vi "get Rx Packet Error.vi"(8 "error in (no error)":errorcluster, 10 "error":u8, 11 "protocol_version":i32) -> (0 "error out":errorcluster, 3 "function return":string)   [LabVIEW 2022 SP3, in "dxl.lvlib"]
doc: "WINDECLSPEC const char *getRxPacketError (int protocol_version, uint8_t error);"
uses:
  dxl.lvlib
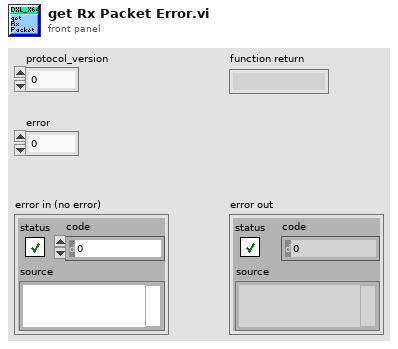
[diagram p1: front panel]
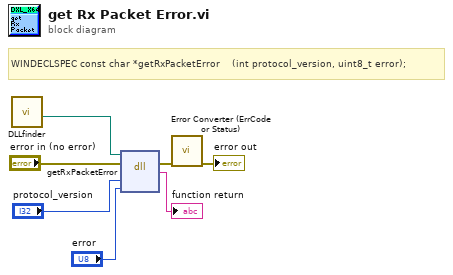
[diagram p0: block diagram]
diagram:
  # "WINDECLSPEC const char *getRxPacketError    (int protocol_version, uint8_t error);"
  n1 = call "DLLfinder.vi"() -> ("File Path"=w1:path)  [unwired: 11 in]
  n2 = dll-call lib="C:/EnFlo_Software/ADAM Serial/Instrument drivers/Dynamixel/2nd attempt/Library/dxl_x64_c.*" fn="getRxPacketError"(path in=w1, error in="error in (no error)", "protocol_version"="protocol_version", "error"="error") -> (error out=w3:errorcluster, "return type"=→"function return":string)  [unwired: 3 in, 1 out]
  n3 = call "Error Converter (ErrCode or Status).vi"("error in (no error)"=w3) -> ("error out"=→"error out":errorcluster)  [unwired: 10 in]
